vi "Rinocloud_children_JSON_parsing.vi"(3 "error in (no error)":errorcluster, 5 "JSON string":string) -> (0 "error out":errorcluster, 2 "metadata array":T1(array[cluster]))   [LabVIEW 2011, in "Rinocloud Library.lvlib"]
uses:
  Rinocloud Library.lvlib
  i3 JSON/i3-json.lvlib
  i3 JSON/JSON Parsing/Get Object Parameter Files/Get Object Parameter - Numeric.vi
  i3 JSON/JSON Parsing/Get Object Parameter Files/Get Object Parameter - String.vi
  i3 JSON/JSON Parsing/Get Object Parameter Files/Get Object Parameter - Array.vi
  i3 JSON/JSON Parsing/Get Array Value at Index Files/Get Array Value at Index - Array.vi
  i3 JSON/JSON Parsing/Get Array Value at Index Files/Get Array Value at Index - String.vi
  i3 JSON/JSON Parsing/Get Object Parameter Files/Get Object Parameter - Object.vi
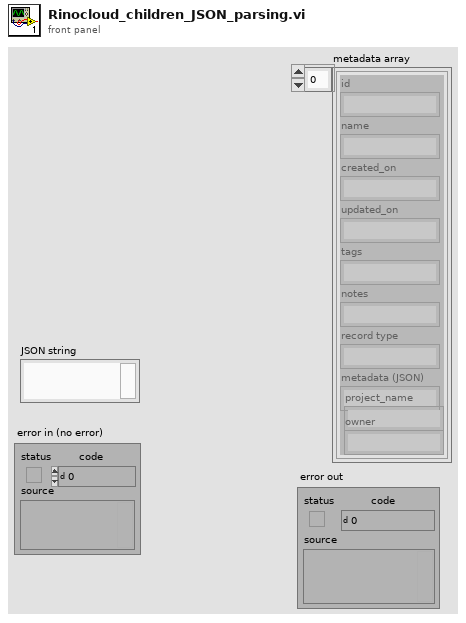
[diagram p1: front panel]
types:
  T1 = cluster{"id":string, "name":string, "created_on":string, "updated_on":string, "tags":string, "notes":string, "record type":string, "metadata (JSON)":string, "project_name":string, "owner":string}[]
  T2 = cluster{"id":string, "name":string, "created_on":string, "updated_on":string, "tags":string, "notes":string, "record type":string, "metadata (JSON)":string, "projec_name":string, "user":string}[]
  T3 = cluster{"id":string, "name":string, "created_on":string, "updated_on":string, "tags":string, "notes":string, "record type":string, "metadata (JSON)":string, "projec_name":string, "user":string}
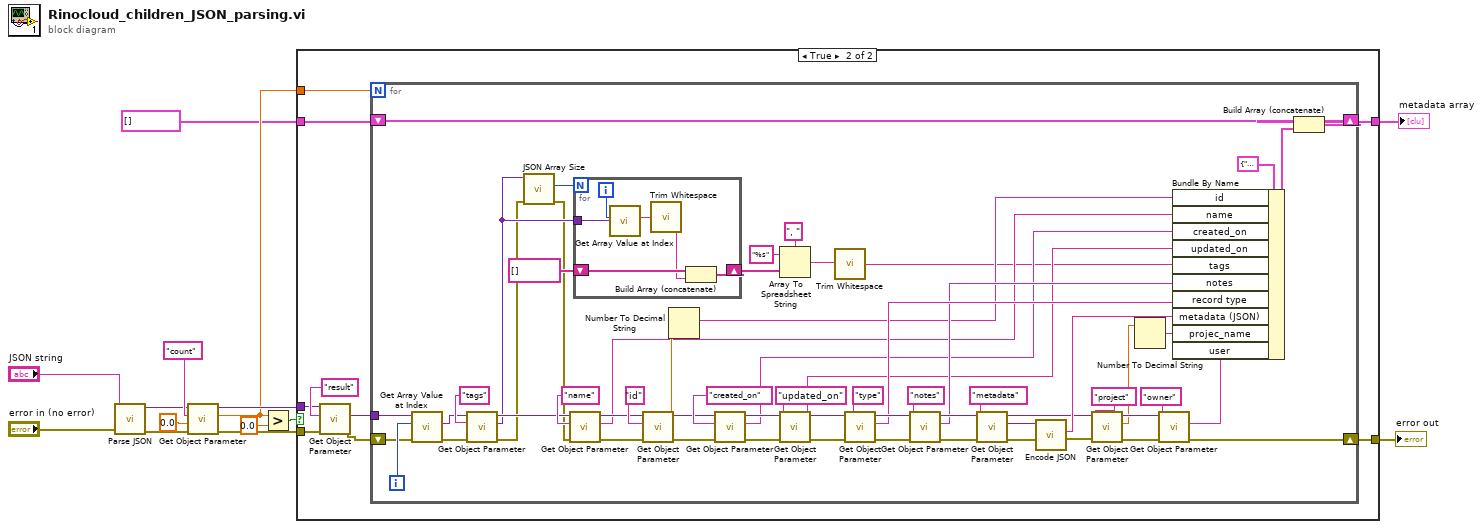
[diagram p0: block diagram]
diagram:
  n1 = call "Parse JSON.vi"("error in (no error)"="error in (no error)", "JSON String"="JSON string") -> ("error out"=w10:errorcluster, "JSON Tree"=w8:variant)  [unwired: 6 in, 2 out]
  n2 = call-poly "Get Object Parameter.vi"("error in (no error)"=w10, "Default Value if JSON Null"=0.0, "Parameter Name"="count", "JSON Tree In (JSON Object)"=w8) -> ("error out"=w9:errorcluster, "Double Value"=w3:dbl, "JSON Tree Out Passthrough"=w7:variant)  [unwired: 4 in, 1 out]
  n3 = Greater?(x=w3, y=0.0) -> (0:w4:bool)
  n4 = case shown="True" w4 {
    tunnel: w9 -> [w15 w24]
    tunnel: w7 -> [_ w23]
    tunnel: w3 -> [_ w22]
    tunnel: [w15 w19] -> w13
    tunnel: [w16 w18] -> w2
    tunnel: T2 [] ("metadata array 2") -> [w16 w17]
    frame False {
    }
    frame True {
      n5 = call-poly "Get Object Parameter.vi"("error in (no error)"=w24, "Parameter Name"="result", "JSON Tree In (JSON Object)"=w23) -> ("error out"=w20:errorcluster, "JSON Array"=w21:variant)  [unwired: 5 in, 2 out]
      n6 = for {
        N: w22 -> [_]
        tunnel: w21 -> [w83]
        shift-right: [w32] -> w19
        shift-left: w20 -> [w77]
        shift-right: [w43] -> w18
        shift-left: w17 -> [w42]
        i -> [w84]
        n7 = call-poly "Get Array Value at Index.vi"("error in (no error)"=w77, "Index"=w84, "JSON Tree In (JSON Array)"=w83) -> ("error out"=w55:errorcluster, "JSON Array"=w40:variant)  [unwired: 5 in, 2 out]
        n8 = call-poly "Get Object Parameter.vi"("error in (no error)"=w55, "Parameter Name"="tags", "JSON Tree In (JSON Object)"=w40) -> ("error out"=w53:errorcluster, "JSON Array"=w54:variant, "JSON Tree Out Passthrough"=w56:variant)  [unwired: 5 in, 1 out]
        n9 = call "JSON Array Size.vi"("error in (no error)"=w53, "JSON Tree In (JSON Array)"=w54) -> ("error out"=w52:errorcluster, "Array Size"=w62:i32)  [unwired: 7 in, 1 out]
        n10 = call-poly "Get Object Parameter.vi"("error in (no error)"=w52, "Parameter Name"="name", "JSON Tree In (JSON Object)"=w56) -> ("error out"=w76:errorcluster, "String Value"=w41:string, "JSON Tree Out Passthrough"=w81:variant)  [unwired: 5 in, 1 out]
        n11 = for {
          N: w62 -> [_]
          tunnel: w54 -> [w91]
          shift-right: [w89] -> w58
          shift-left: string[] [] ("Tags 2") -> [w90]
          i -> [w88]
          n12 = call-poly "Get Array Value at Index.vi"("Index"=w88, "JSON Tree In (JSON Array)"=w91) -> ("String Value"=w87:string)  [unwired: 6 in, 3 out]
          n13 = call <vilib>:"Trim Whitespace.vi"("string"=w87) -> ("trimmed string"=w86:string)  [unwired: 1 in]
          n14 = Build Array (concatenate)(w90, w86) -> (w89:string[])
        }
        n15 = call-poly "Get Object Parameter.vi"("error in (no error)"=w76, "Parameter Name"="id", "JSON Tree In (JSON Object)"=w81) -> ("error out"=w66:errorcluster, "Double Value"=w63:dbl, "JSON Tree Out Passthrough"=w67:variant)  [unwired: 5 in, 1 out]
        n16 = Number To Decimal String(number=w63) -> (decimal integer string=w44:string)  [unwired: 1 in]
        n17 = call-poly "Get Object Parameter.vi"("error in (no error)"=w66, "Parameter Name"="created_on", "JSON Tree In (JSON Object)"=w67) -> ("error out"=w64:errorcluster, "String Value"=w45:string, "JSON Tree Out Passthrough"=w65:variant)  [unwired: 5 in, 1 out]
        n18 = Array To Spreadsheet String(delimiter (Tab)=", ", array=w58, 3:"%s" ("format string")) -> (spreadsheet string=w39:string)
        n19 = call-poly "Get Object Parameter.vi"("error in (no error)"=w64, "Parameter Name"="updated_on", "JSON Tree In (JSON Object)"=w65) -> ("error out"=w75:errorcluster, "String Value"=w46:string, "JSON Tree Out Passthrough"=w78:variant)  [unwired: 5 in, 1 out]
        n20 = call <vilib>:"Trim Whitespace.vi"("string"=w39) -> ("trimmed string"=w38:string)  [unwired: 1 in]
        n21 = call-poly "Get Object Parameter.vi"("error in (no error)"=w75, "Parameter Name"="type", "JSON Tree In (JSON Object)"=w78) -> ("error out"=w50:errorcluster, "String Value"=w48:string, "JSON Tree Out Passthrough"=w51:variant)  [unwired: 5 in, 1 out]
        n22 = call-poly "Get Object Parameter.vi"("error in (no error)"=w50, "Parameter Name"="notes", "JSON Tree In (JSON Object)"=w51) -> ("error out"=w70:errorcluster, "String Value"=w47:string, "JSON Tree Out Passthrough"=w73:variant)  [unwired: 5 in, 1 out]
        n23 = call-poly "Get Object Parameter.vi"("error in (no error)"=w70, "Parameter Name"="metadata", "JSON Tree In (JSON Object)"=w73) -> ("error out"=w69:errorcluster, "JSON Object"=w71:variant, "JSON Tree Out Passthrough"=w31:variant)  [unwired: 5 in, 1 out]
        n24 = call "Encode JSON.vi"("error in (no error)"=w69, "JSON Tree"=w71) -> ("error out"=w33:errorcluster, "String"=w49:string)  [unwired: 4 in]
        n25 = call-poly "Get Object Parameter.vi"("error in (no error)"=w33, "Parameter Name"="project", "JSON Tree In (JSON Object)"=w31) -> ("error out"=w37:errorcluster, "Double Value"=w26:dbl, "JSON Tree Out Passthrough"=w35:variant)  [unwired: 5 in, 1 out]
        n26 = Number To Decimal String(number=w26) -> (decimal integer string=w27:string)  [unwired: 1 in]
        n27 = call-poly "Get Object Parameter.vi"("error in (no error)"=w37, "Parameter Name"="owner", "JSON Tree In (JSON Object)"=w35) -> ("error out"=w32:errorcluster, "String Value"=w29:string)  [unwired: 5 in, 2 out]
        n28 = Bundle By Name(cluster=T3 {"id"="", "name"="", "created_on"="", "updated_on"="", "tags"="", "notes"="", "record type"="", "metadata (JSON)"="", "projec_name"="", "user"=""} ("metadata 2"), "id"=w44, "name"=w41, "created_on"=w45, "updated_on"=w46, "tags"=w38, "notes"=w47, "record type"=w48, "metadata (JSON)"=w49, "projec_name"=w27, "user"=w29) -> (w28:T3)
        n29 = Build Array (concatenate)(w42, w28) -> (w43:T2)
      }
    }
  }
  "error out" <- w13
  "metadata array" <- w2
